vi "Emballage_BDD_lectureSQL_Depuis_SN_PRODUIT.vi"(4 "ID_ARTICLE?":bool, 5 "Where (Champs:SN_PRODUIT)":string[](array[string])=["SN_PRODUIT"], 6 "order by ... DESC":string="DATE_EMBALLAGE", 7 "Where (Like/=)":string="=", 8 "Error in":errorcluster caption="Error in (no error)", 9 "Colonnes":string[](array[string])=["SN_PRODUIT\n", "DATE_EMBALLAGE\n", "ID_UTILISATEUR_GPAO\n", "NO_CDEVAL\n", "NO_DU_CARTON\n", "NO_RETOUR_CLIENT\n", "ID_ARTICLE_GPAO"], 10 "Where (Valeur)":string[](array[string]), 11 "Table (PRODUIT_EMBALLAGE)":string="PRODUIT_EMBALLAGE") -> (0 "Error out":errorcluster, 2 "Erreur de  comunication":bool, 3 "Donnees":string[][](array[string]))   [LabVIEW 2020]
uses:
  Modules/FS/60_FS_Controles/60_FS_SetGet.ctl
  <vilib>/addons/database/Connection.llb/DB Tools Open Connec (Path).vi
  <vilib>/addons/database/Connection.llb/Conn Execute.vi
  <vilib>/addons/database/Recordset.llb/Rec Fetch Recordset Data (R).vi
  <vilib>/addons/database/Recordset.llb/Rec Destroy - Connection.vi
  <vilib>/addons/database/NI_Database_API.lvlib
panel:
  # "6"
  # "0"
  # "2"
  # "3"
  # "4"
  # "5"
  # "1"
  # "0: SN_PRODUIT\n1: DATE_EMBALLAGE\n2: ID_UTILISATEUR_GPAO\n3: NO_CDEVAL\n4: NO_DU_CARTON\n5: NO_RETOUR_CLIENT\n6: ID_ARTICLE_GPAO"
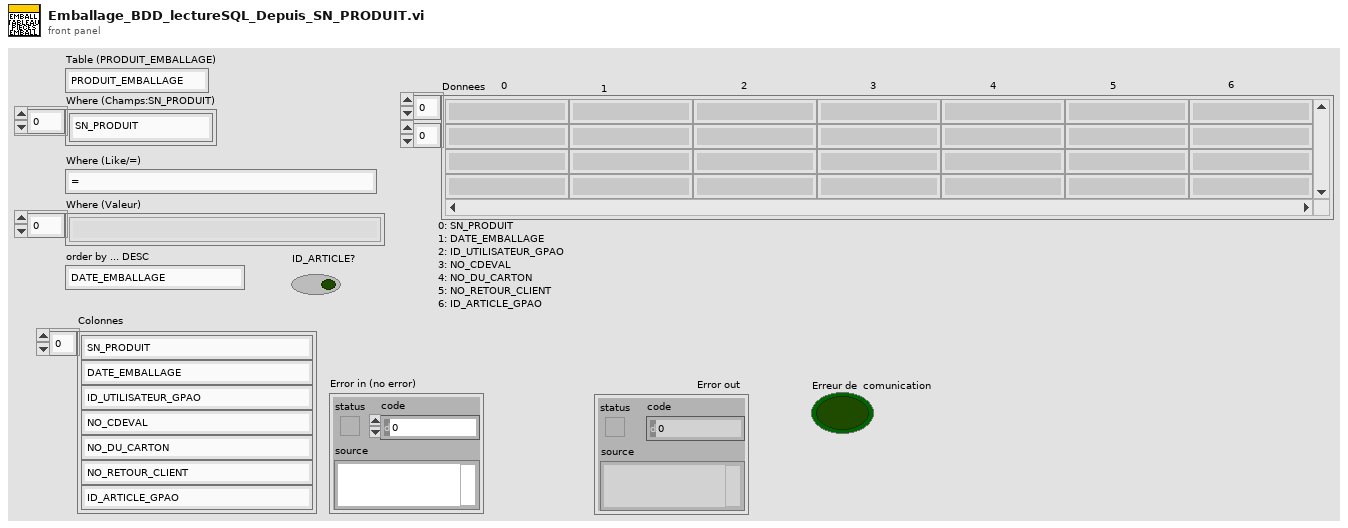
[diagram p1: front panel]
types:
  T1 = typedef "60_FS_SetGet.ctl" = enum16{"set", "get"}
  T2 = typedef "60_FS_CLT_Chemins.ctl" = cluster{"Racine_local":path, "Racine_reseau":path, "Racine_Support_Application":path, "Fichier_Journalisation":path, "Connexion_BDD_VSX":path, "Connexion_BDD_PLZ":path}
  T3 = typedef "NI_Database_API.lvlib/Conn ObjectReference.ctl" = refnum<k1>
  T4 = typedef "NI_Database_API.lvlib/Rec ObjectReference.ctl" = refnum<k1>
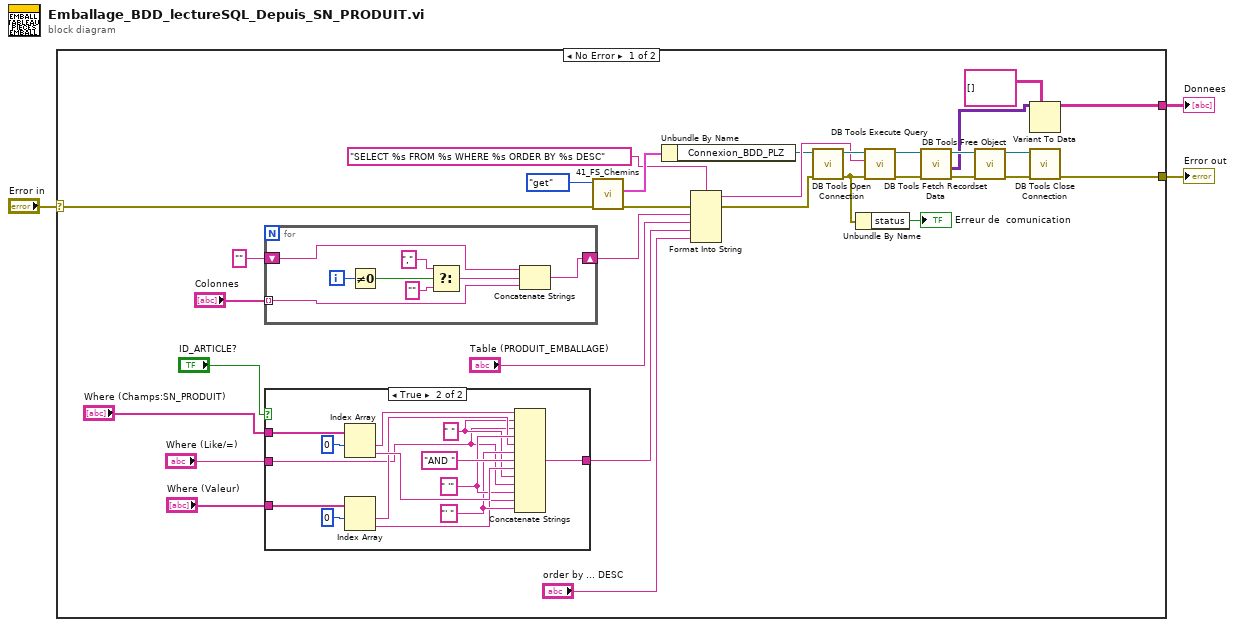
[diagram p0: block diagram]
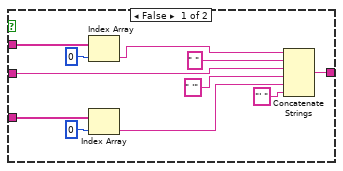
[diagram p2: hidden frame]
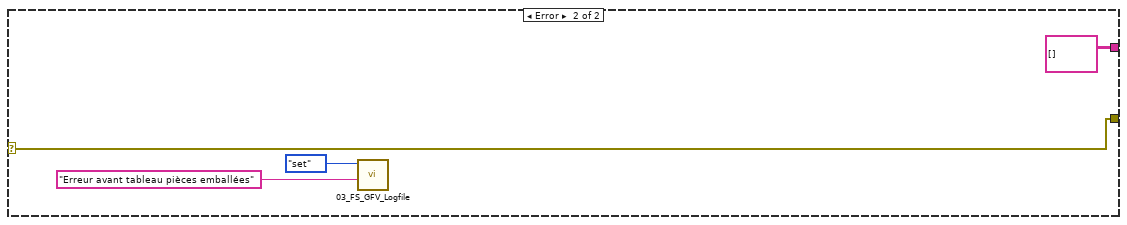
[diagram p3: hidden frame]
diagram:
  n1 = case shown="No Error" "Error in" {
    selector: "Error in" -> [w26 w71]
    tunnel: [w25 w71] -> w2
    tunnel: [w18 string[][] [] ("Liste des champs à lire 2")] -> w1
    frame No Error {
      n2 = for {
        tunnel: "Colonnes" -> [w66] mode=indexing
        shift-right: [w67] -> w15
        shift-left: "" -> [w65]
        i -> [w64]
        n3 = Not Equal To 0?(x=w64) -> (x != 0?=w63:bool)
        n4 = Select(t="," ("cas vrai"), s=w63, f="") -> (s? t:f=w62:string)
        n5 = Concatenate Strings(w65, w62, w66) -> (w67:string)
      }
      n6 = case shown="True" "ID_ARTICLE?" {
        tunnel: [w45 w52] -> w5
        tunnel: "Where (Champs:SN_PRODUIT)" -> [w42 w57]
        tunnel: "Where (Valeur)" -> [w36 w50]
        tunnel: "Where (Like/=)" -> [w38 w46]
        frame False {
          n7 = Index Array(array=w42, index=0 ("indice")) -> (element=w40:string)
          n8 = Index Array(array=w36, index=0 ("indice")) -> (element=w35:string)
          n9 = Concatenate Strings(w40, " " ("chaîne"), w38, " '" ("chaîne"), w35, "' " ("chaîne")) -> (w45:string)
        }
        frame True {
          w47 = " " ("chaîne")
          w53 = "' " ("chaîne")
          w54 = " '" ("chaîne")
          n10 = Index Array(array=w57, index #1=0 ("indice")) -> (element #1=w59:string, element #2=w55:string)  [unwired: 1 in]
          n11 = Index Array(array=w50, index #1=0 ("indice")) -> (element #1=w49:string, element #2=w51:string)  [unwired: 1 in]
          n12 = Concatenate Strings(w59, w47, w46, w54, w49, w53, "AND " ("chaîne"), w55, w47, w46, w54, w51, w53) -> (w52:string)
        }
      }
      n13 = call "41_FS_Chemins.vi"("error in (no error)"=w26, "SetGet"=60_FS_SetGet."get") -> ("error out"=w4:errorcluster, "CLT_Chemins_out"=w30:T2)  [unwired: 8 in]
      n14 = Unbundle By Name(w30) -> ("Connexion_BDD_PLZ"=w11:path)
      n15 = Format Into String(format string="SELECT %s FROM %s WHERE %s ORDER BY %s DESC" ("chaîne de format"), error in=w4, w15, "Table (PRODUIT_EMBALLAGE)", w5, "order by ... DESC") -> (resulting string=w27:string, error out=w31:errorcluster)  [unwired: 1 in]
      n16 = call-poly <vilib>:"DB Tools Open Connection.vi"("error in (no error)"=w31, "connection information"=w11) -> ("error out"=w13:errorcluster, "connection reference"=w32:T3)  [unwired: 6 in]
      n17 = Unbundle By Name(w13) -> ("status"=→"Erreur de  comunication":bool)
      n18 = call-poly <vilib>:"DB Tools Execute Query.vi"("error in (no error)"=w13, "SQL query"=w27, "connection reference"=w32) -> ("error out"=w24:errorcluster, "recordset reference"=w22:T4)  [unwired: 5 in]
      n19 = call-poly <vilib>:"DB Tools Fetch Recordset Data.vi"("error in (no error)"=w24, "recordset reference"=w22) -> ("error out"=w23:errorcluster, "recordset data"=w20:variant[][], "recordset reference out"=w21:T4)  [unwired: 3 in]
      n20 = call-poly <vilib>:"DB Tools Free Object.vi"("error in (no error)"=w23, "recordset reference"=w21) -> ("error out"=w34:errorcluster, "connection reference"=w33:T3)  [unwired: 8 in]
      n21 = Variant To Data(type=string[][] [] ("Liste des champs à lire 2"), Variant=w20) -> (data=w18:string[][])  [unwired: 1 in, 1 out]
      n22 = call <vilib>:"DB Tools Close Connection.vi"("error in (no error)"=w34, "connection reference"=w33) -> ("error out"=w25:errorcluster)  [unwired: 5 in]
    }
    frame Error {
      n23 = call "03_FS_GFV_Logfile.vi"("Chaîne"="Erreur avant tableau pièces emballées", "States"=60_FS_SetGet."set") -> ()  [unwired: 8 in, 2 out]
    }
  }
  "Error out" <- w2
  "Donnees" <- w1
